vi "표지판 가공(동적).vi"(0 "Image 2":T2, 1 "Classifier Session (optional)":T1, 2 "File Path":path=path "C:/Users/김남규/Desktop/남규/Vision/Particle Classification 최종/동적 장애물 Dark.clf", 3 "Paramaters":T4={"Preprocessing Options"={"Method"=-1, "Looking for"=0, "Threshold Range"={"Lower value"=0.0, "Upper value"=45.0}, "Threshold Limits"={"Lower value"=0.0, "Upper value"=0.0}, "Reject Border"=FALSE, "# of Erosions"=0, "Kernel Size"={"Lower value"=0, "Upper value"=0}, "Deviation Factor"=0.0}, "Nearest Neighbor Options"={"Method"=0, "Metric"=0, "k"=0}, "Particle Options"={"Scale Dependant"=FALSE, "Scale Factor"=0.0, "Symmetry Dependant"=FALSE, "Symmetry Factor"=0.0}} {"Preprocessing Options"."Deviation Factor" min=0.0; "Preprocessing Options"."Threshold Limits"."Upper value" format="%.2f"; "Preprocessing Options"."Threshold Limits"."Lower value" format="%.2f"; "Preprocessing Options"."Threshold Range"."Upper value" format="%.2f"; "Preprocessing Options"."Threshold Range"."Lower value" format="%.2f"; "Preprocessing Options"."# of Erosions" min=0; "Preprocessing Options"."Method" items=["Manual Threshold"=-1, "-"=-2, "Auto Threshold: Clustering"=0, "Auto Threshold: Entropy"=1, "Auto Threshold: Metric"=2, "Auto Threshold: Moments"=3, "Auto Threshold: Inter-class Variance"=4, "--"=-3, "Local Threshold: Niblack"=5, "Local Threshold: BG Correction"=6]; "Preprocessing Options"."Looking for" items=["Bright Objects", "Dark Objects"]; "Nearest Neighbor Options"."Method" items=["Nearest Neighbor", "K Nearest Neighbor", "Minimum Mean Distance"]; "Nearest Neighbor Options"."Metric" items=["Maximum", "Sum", "Euclidean"]; "Nearest Neighbor Options"."k" min=3}, 5 "ROI Descriptor (Particle Classification 1)":T5={"Global Rectangle"=[750, 250, 1250, 750], "Contours"=[{"ID"=enum."External", "Type"=3, "Coordinates"=[693, 212, 1098, 745]}]} {"Contours"."Type" items=["No Selection", "Point", "Line", "Rectangle", "Oval", "Polygon", "Freehand Region", "Annulus", "Unused2", "Unused3", "Broken Line", "Freehand Line", "Rotated Rectangle"]}) -> (4 "주차냐":bool, 6 "Classifier Session (dup)":T1, 9 "error out":errorcluster, 10 "Image":T2(plugin-control))   [LabVIEW 2016]
uses:
  <vilib>/vision/Classification.llb/IMAQ Classifier Nearest Neighbor options.ctl
  <vilib>/vision/Classification.llb/IMAQ Classifier Session.ctl
  <vilib>/vision/Image Controls.llb/IMAQ Image.ctl
  <vilib>/vision/NI_Vision_Development_Module.lvlib
panel:
  out "Identification Score":sgl
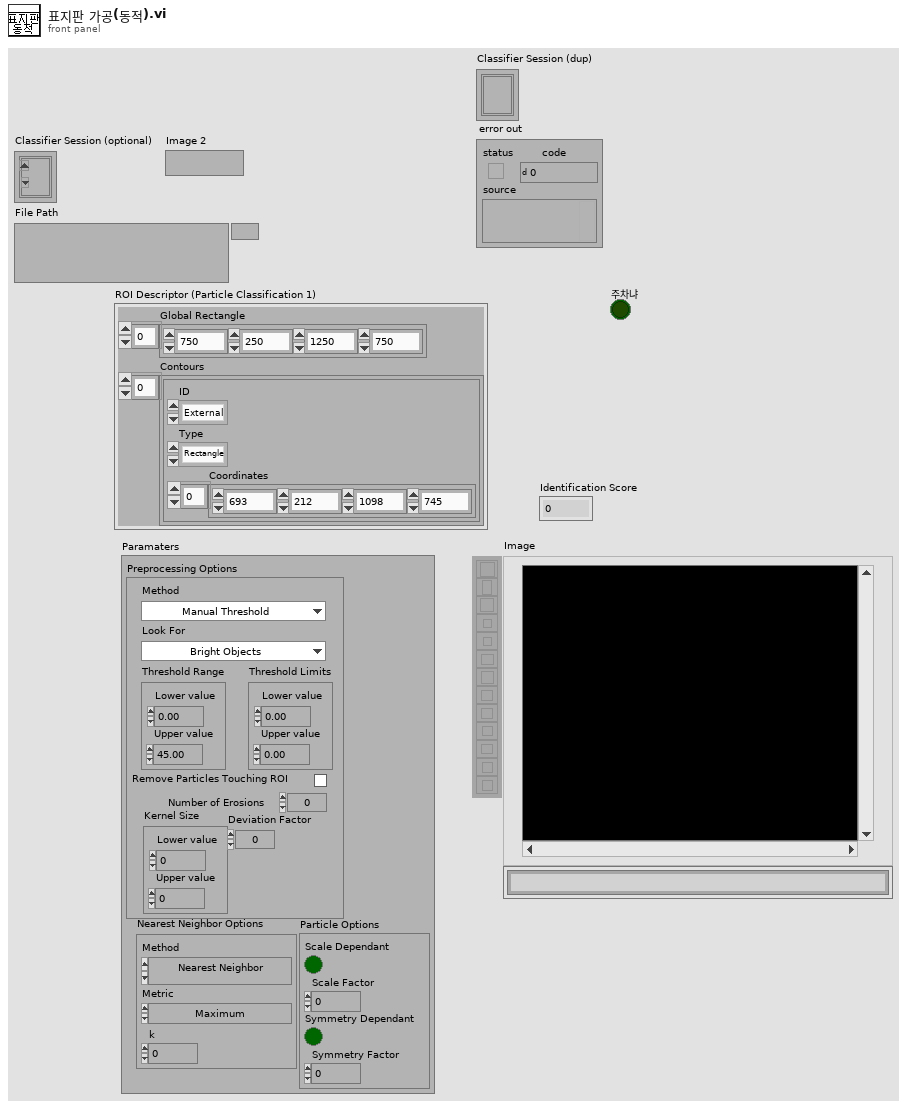
[diagram p1: front panel]
types:
  T1 = typedef "IMAQ Classifier Session.ctl" = refnum<k1>
  T2 = typedef "IMAQ Image.ctl" = refnum<image>
  T3 = typedef "IMAQ Classifier Nearest Neighbor options.ctl" = cluster{"Method":i32, "Metric":i32, "k":i32}
  T4 = cluster{"Preprocessing Options":cluster{"Method":i32, "Looking for":i32, "Threshold Range":cluster{"Lower value":sgl, "Upper value":sgl}, "Threshold Limits":cluster{"Lower value":sgl, "Upper value":sgl}, "Reject Border":bool, "# of Erosions":i32, "Kernel Size":cluster{"Lower value":i32, "Upper value":i32}, "Deviation Factor":dbl}, "Nearest Neighbor Options":T3, "Particle Options":cluster{"Scale Dependant":bool, "Scale Factor":sgl, "Symmetry Dependant":bool, "Symmetry Factor":sgl}}
  T5 = cluster{"Global Rectangle":i32[], "Contours":cluster{"ID":enum32{"External", "Internal"}, "Type":u32, "Coordinates":i32[]}[]}
  T6 = cluster{"Classification Score":sgl, "Identification Score":sgl}
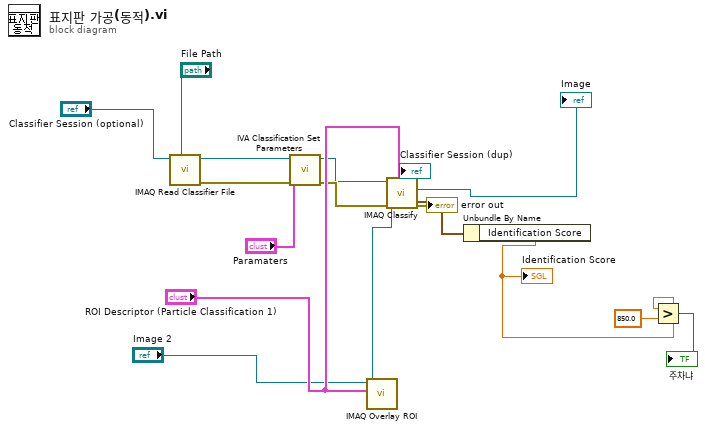
[diagram p0: block diagram]
diagram:
  n1 = call "IMAQ Read Classifier File"("File Path"="File Path", "Classifier Session (optional)"="Classifier Session (optional)") -> ("error out"=w13:errorcluster, "Classifier Session"=w14:T1)  [unwired: 5 in, 3 out]
  n2 = call <vilib>:"IVA Classification Set Parameters.vi"("error in"=w13, "Paramaters"="Paramaters", "Classifier Session In"=w14) -> ("error out"=w12:errorcluster, "Classifier Session Out"=w8:T1)  [unwired: 7 out]
  n3 = call "IMAQ Overlay ROI"("ROI Descriptor"="ROI Descriptor (Particle Classification 1)", "Image"="Image 2") -> ("Image Out"=w17:T2)  [unwired: 8 in, 1 out]
  n4 = call "IMAQ Classify"("ROI Descriptor"="ROI Descriptor (Particle Classification 1)", "error in (no error)"=w12, "Image"=w17, "Classifier Session"=w8) -> ("error out"=→"error out":errorcluster, "Image (dup)"=→"Image":T2, "Classifier Session (dup)"=→"Classifier Session (dup)":T1, "Scores"=w15:T6)  [unwired: 2 in, 2 out]
  n5 = Unbundle By Name(w15) -> ("Identification Score"=w11:sgl)
  "Identification Score" <- w11
  n6 = Greater?(x=w11, y=sgl 850.0) -> (0:→"주차냐":bool)
